vi "TCPclientpython.vi"(6 "Input Command":string="Mock TE UVa test coil\r\nQCV3598277979.csv\r\nUnused\r\nNMRave.csv\r\nUnused\r\nTune2.csv\r\n\r\n\r\n\r\n\r\n35982.0000\r\n87350.1529\r\n  213.0000\r\n    0.0020\r\n  401.0000\r\n    1.0000\r\n   23.0000\r\n    3.2790\r\n    1.4760\r\n    1.3028\r\n    8.3950\r\n   -0.3883\r\n    1.0000\r\n    1.0000\r\n    1.0000\r\n    1.0000\r\n    0.0000\r\n    0.0129\r\n    2.0000\r\n  212.9745\r\n    0.0000\r\n    0.0000\r\n    4.0000\r\n    2.1333\r\n   33.8900\r\n    0.0011\r\n    0.0009\r\n    0.0008\r\n    0.0008\r\n    0.0008\r\n    0.0008\r\n    0.0005\r\n    0.0006\r\n    0.0005\r\n    0.0006\r\n    0.0006\r\n    0.0006\r\n    0.0006\r\n    0.0005\r\n    0.0003\r\n    0.0003\r\n   -0.0000\r\n   -0.0000\r\n    0.0002\r\n    0.0002\r\n    0.0002\r\n   -0.0000\r\n   -0.0000\r\n   -0.0000\r\n   -0.0000\r\n   -0.0002\r\n   -0.0000\r\n   -0.0002\r\n   -0.0002\r\n   -0.0003\r\n   -0.0002\r\n   -0.0002\r\n   -0.0003\r\n   -0.0003\r\n   -0.0005\r\n   -0.0003\r\n   -0.0005\r\n   -0.0003\r\n   -0.0005\r\n   -0.0005\r\n   -0.0006\r\n   -0.0006\r\n   -0.0008\r\n   -0.0008\r\n   -0.0008\r\n   -0.0008\r\n   -0.0008\r\n   -0.0008\r\n   -0.0008\r\n   -0.0009\r\n   -0.0009\r\n   -0.0011\r\n   -0.0012\r\n   -0.0011\r\n   -0.0011\r\n   -0.0011\r\n   -0.0012\r\n   -0.0012\r\n   -0.0012\r\n   -0.0012\r\n   -0.0014\r\n   -0.0014\r\n   -0.0012\r\n   -0.0014\r\n   -0.0014\r\n   -0.0015\r\n   -0.0015\r\n   -0.0017\r\n   -0.0017\r\n   -0.0017\r\n   -0.0017\r\n   -0.0017\r\n   -0.0017\r\n   -0.0018\r\n   -0.0018\r\n   -0.0017\r\n   -0.0018\r\n   -0.0017\r\n   -0.0017\r\n   -0.0020\r\n   -0.0020\r\n   -0.0018\r\n   -0.0021\r\n   -0.0023\r\n   -0.0021\r\n   -0.0024\r\n   -0.0023\r\n   -0.0021\r\n   -0.0023\r\n   -0.0023\r\n   -0.0021\r\n   -0.0021\r\n   -0.0020\r\n   -0.0021\r\n   -0.0021\r\n   -0.0023\r\n   -0.0024\r\n   -0.0024\r\n   -0.0023\r\n   -0.0024\r\n   -0.0024\r\n   -0.0026\r\n   -0.0027\r\n   -0.0024\r\n   -0.0027\r\n   -0.0026\r\n   -0.0026\r\n   -0.0024\r\n   -0.0026\r\n   -0.0027\r\n   -0.0027\r\n   -0.0027\r\n   -0.0026\r\n   -0.0026\r\n   -0.0026\r\n   -0.0029\r\n   -0.0029\r\n   -0.0031\r\n   -0.0029\r\n   -0.0031\r\n   -0.0029\r\n   -0.0027\r\n   -0.0027\r\n   -0.0027\r\n   -0.0029\r\n   -0.0027\r\n   -0.0031\r\n   -0.0031\r\n   -0.0032\r\n   -0.0032\r\n   -0.0031\r\n   -0.0032\r\n   -0.0031\r\n   -0.0031\r\n   -0.0032\r\n   -0.0031\r\n   -0.0031\r\n   -0.0031\r\n   -0.0032\r\n   -0.0035\r\n   -0.0032\r\n   -0.0032\r\n   -0.0032\r\n   -0.0031\r\n   -0.0031\r\n   -0.0031\r\n   -0.0031\r\n   -0.0032\r\n   -0.0031\r\n   -0.0032\r\n   -0.0034\r\n   -0.0035\r\n   -0.0035\r\n   -0.0034\r\n   -0.0034\r\n   -0.0032\r\n   -0.0032\r\n   -0.0034\r\n   -0.0032\r\n   -0.0032\r\n   -0.0034\r\n   -0.0035\r\n   -0.0032\r\n   -0.0032\r\n   -0.0035\r\n   -0.0034\r\n   -0.0032\r\n   -0.0031\r\n   -0.0031\r\n   -0.0032\r\n   -0.0031\r\n   -0.0029\r\n   -0.0027\r\n   -0.0027\r\n   -0.0027\r\n   -0.0027\r\n   -0.0026\r\n   -0.0024\r\n   -0.0020\r\n   -0.0017\r\n   -0.0011\r\n   -0.0003\r\n    0.0012\r\n    0.0040\r\n    0.0085\r\n    0.0117\r\n    0.0110\r\n    0.0087\r\n    0.0082\r\n    0.0095\r\n    0.0107\r\n    0.0082\r\n    0.0034\r\n   -0.0000\r\n   -0.0015\r\n   -0.0026\r\n   -0.0032\r\n   -0.0032\r\n   -0.0035\r\n   -0.0037\r\n   -0.0038\r\n   -0.0040\r\n   -0.0038\r\n   -0.0038\r\n   -0.0040\r\n   -0.0040\r\n   -0.0038\r\n   -0.0038\r\n   -0.0038\r\n   -0.0038\r\n   -0.0038\r\n   -0.0038\r\n   -0.0040\r\n   -0.0041\r\n   -0.0040\r\n   -0.0041\r\n   -0.0040\r\n   -0.0040\r\n   -0.0038\r\n   -0.0038\r\n   -0.0038\r\n   -0.0038\r\n   -0.0040\r\n   -0.0041\r\n   -0.0040\r\n   -0.0038\r\n   -0.0037\r\n   -0.0037\r\n   -0.0038\r\n   -0.0037\r\n   -0.0038\r\n   -0.0037\r\n   -0.0034\r\n   -0.0034\r\n   -0.0037\r\n   -0.0035\r\n   -0.0034\r\n   -0.0032\r\n   -0.0031\r\n   -0.0027\r\n   -0.0020\r\n   -0.0008\r\n   -0.0002\r\n   -0.0008\r\n   -0.0012\r\n   -0.0011\r\n   -0.0003\r\n   -0.0000\r\n   -0.0009\r\n   -0.0023\r\n   -0.0029\r\n   -0.0034\r\n   -0.0035\r\n   -0.0035\r\n   -0.0037\r\n   -0.0037\r\n   -0.0037\r\n   -0.0035\r\n   -0.0037\r\n   -0.0037\r\n   -0.0035\r\n   -0.0034\r\n   -0.0034\r\n   -0.0037\r\n   -0.0037\r\n   -0.0035\r\n   -0.0034\r\n   -0.0032\r\n   -0.0034\r\n   -0.0034\r\n   -0.0034\r\n   -0.0034\r\n   -0.0032\r\n   -0.0032\r\n   -0.0032\r\n   -0.0031\r\n   -0.0029\r\n   -0.0027\r\n   -0.0027\r\n   -0.0026\r\n   -0.0024\r\n   -0.0026\r\n   -0.0026\r\n   -0.0027\r\n   -0.0027\r\n   -0.0026\r\n   -0.0026\r\n   -0.0027\r\n   -0.0029\r\n   -0.0029\r\n   -0.0029\r\n   -0.0029\r\n   -0.0027\r\n   -0.0024\r\n   -0.0020\r\n   -0.0009\r\n    0.0002\r\n    0.0012\r\n    0.0009\r\n   -0.0000\r\n   -0.0000\r\n    0.0008\r\n    0.0011\r\n    0.0005\r\n   -0.0009\r\n   -0.0020\r\n   -0.0023\r\n   -0.0024\r\n   -0.0026\r\n   -0.0026\r\n   -0.0026\r\n   -0.0026\r\n   -0.0026\r\n   -0.0026\r\n   -0.0024\r\n   -0.0024\r\n   -0.0023\r\n   -0.0023\r\n   -0.0024\r\n   -0.0026\r\n   -0.0026\r\n   -0.0023\r\n   -0.0023\r\n   -0.0023\r\n   -0.0023\r\n   -0.0021\r\n   -0.0018\r\n   -0.0021\r\n   -0.0021\r\n   -0.0021\r\n   -0.0021\r\n   -0.0021\r\n   -0.0021\r\n   -0.0020\r\n   -0.0018\r\n   -0.0018\r\n   -0.0017\r\n   -0.0018\r\n   -0.0020\r\n   -0.0017\r\n   -0.0015\r\n   -0.0015\r\n   -0.0015\r\n   -0.0015\r\n   -0.0015\r\n   -0.0014\r\n   -0.0015\r\n   -0.0018\r\n   -0.0015\r\n   -0.0014\r\n   -0.0012\r\n   -0.0009\r\n   -0.0011\r\n   -0.0009\r\n   -0.0008\r\n   -0.0009\r\n   -0.0008\r\n   -0.0008\r\n   -0.0011\r\n   -0.0012\r\n   -0.0009\r\n   -0.0008\r\n   -0.0008\r\n   -0.0008\r\n   -0.0006\r\n   -0.0005\r\n   -0.0005\r\n   -0.0003\r\n   -0.0002\r\n   -0.0002\r\n   -0.0002\r\n   -0.0003\r\n   -0.0002\r\n   -0.0003\r\n   -0.0002\r\n   -0.0002\r\n   -0.0002\r\n   -0.0002\r\n   -0.0000\r\n   -0.0000\r\n   -0.0000\r\n   -0.0000\r\n   -0.0000\r\n   -0.0000\r\n   -0.0000\r\n    0.0002\r\n    0.0002\r\n    0.0002\r\n    0.0005\r\n    0.0006\r\n    0.0005\r\n    0.0005\r\n    0.0006\r\n    0.0008\r\n    0.0006\r\n    0.0008\r\n    0.0009\r\n    0.0009\r\n    0.0012\r\n    0.0012\r\n    0.0012\r\n") -> (0 "Telnet error":errorcluster={"status"=TRUE, "code"=0, "source"="Telnet Registry.vi [get data]: invalid object 0"}, 2 "Command and Results":string, 3 "Open Connection":string)   [LabVIEW 2018]
doc: "The Telnet Line Client VI uses the Telnet VIs to simulate a simple Telnet Window."
uses:
  Global 2.vi
panel:
  out "Bytes written":i32
  in  "PythonIP":string="127.0.0.1"
  out "First":bool=TRUE
  in  "Port #":i32=10023
  # "Python TCP/IO Routine"
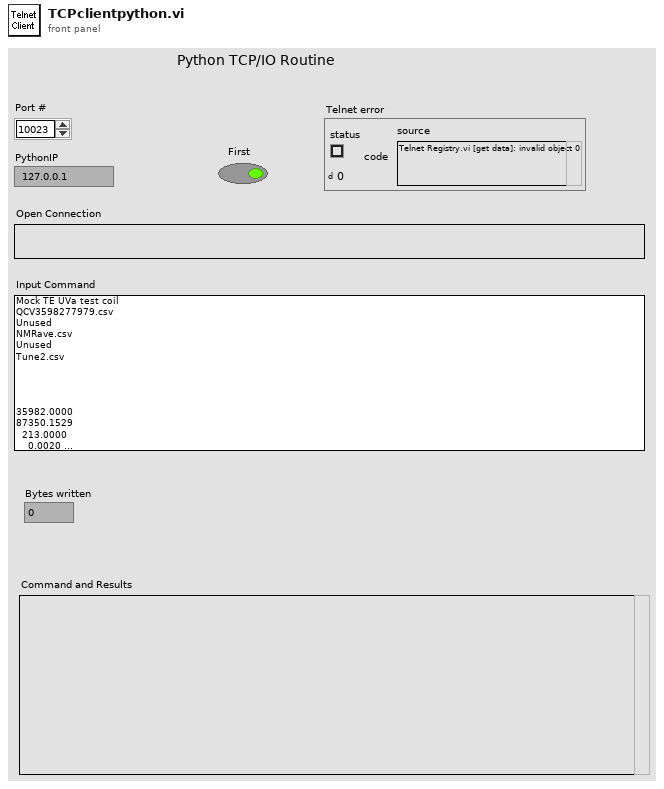
[diagram p1: front panel]
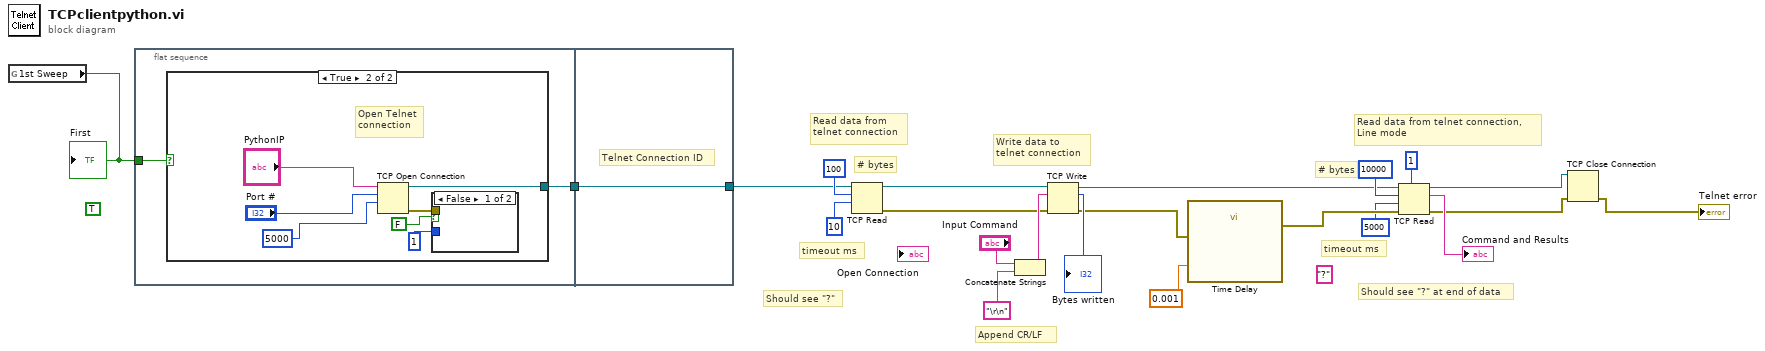
[diagram p0: block diagram]
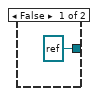
[diagram p2: hidden frame]
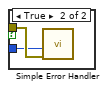
[diagram p3: hidden frame]
diagram:
  (unwired) TRUE
  (unwired) "?"
  # "timeout ms"
  # "# bytes"
  # "Should see \"?\""
  # "Read data from \ntelnet connection"
  # "timeout ms"
  # "# bytes"
  # "Should see \"?\" at end of data"
  # "Read data from telnet connection, \nLine mode"
  # "Append CR/LF"
  # "Write data to \ntelnet connection"
  n1 = global read "Global 2.vi" "1st Sweep"() -> (w11:bool)
  "First" <- w11
  n2 = flat-sequence {
    tunnel: w11 -> [w24]
    tunnel: [w23] -> w10
    tunnel: [w35] -> w9
    tunnel: w10 -> [w35]
    frame #0 {
      n3 = case shown="True" w24 {
        tunnel: [refnum<k5> refnum ("connection ID") w26] -> w23
        frame False {
        }
        frame True {
          # "Open Telnet\nconnection"
          n4 = TCP Open Connection(address="PythonIP", remote port or service name="Port #", timeout ms (60000)=5000) -> (connection ID=w26:refnum<k5>, error out=w30:errorcluster)  [unwired: 2 in]
          n5 = case shown="False" FALSE {
            tunnel: w30 -> [_ w34]
            tunnel: 1 -> [_ w33]
            frame False {
            }
            frame True {
              n6 = call <vilib>:"Simple Error Handler.vi"("type of dialog (OK msg:1)"=w33, "error in (no error)"=w34) -> ()  [unwired: 3 in, 5 out]
            }
          }
        }
      }
    }
    frame #1 {
      # "Telnet Connection ID"
    }
  }
  n7 = TCP Read(connection ID=w9, bytes to read=100, 9:10 ("timeout ms (25000)")) -> (connection ID out=w8:refnum<k5>, error out=w19:errorcluster)  [unwired: 2 in, 1 out]
  n8 = Concatenate Strings("Input Command", "\r\n") -> (w20:string)
  n9 = TCP Write(connection ID=w8, data in=w20, error in (no error)=w19) -> (connection ID out=w4:refnum<k5>, bytes written=→"Bytes written":i32, error out=w12:errorcluster)  [unwired: 1 in]
  n10 = call "Time Delay"("error in (no error)"=w12, "Delay Time (s)"=0.001) -> ("error out"=w7:errorcluster)  [unwired: 9 in]
  n11 = TCP Read(connection ID=w4, bytes to read=10000, error in (no error)=w7, 7:1, 9:5000 ("timeout ms (25000)")) -> (connection ID out=w3:refnum<k5>, data out=→"Command and Results":string, error out=w2:errorcluster)
  n12 = TCP Close Connection(connection ID=w3, error in (no error)=w2) -> (error out=→"Telnet error":errorcluster)  [unwired: 1 in, 1 out]
